vi "Routine.vi"(11 "TEMPLATE Queue in":refnum<class "TEMPLATE Queue.lvclass">) -> (3 "TEMPLATE Queue out":refnum<class "TEMPLATE Queue.lvclass">)   [LabVIEW 2021, in "_Template.lvlib" / "Templates.lvlib" / "TEMPLATE Queue.lvlib" / "TEMPLATE Queue.lvclass"]
uses:
  TEMPLATE Queue.lvclass
  TEMPLATE Queue.lvclass/TEMPLATE Queue.ctl
  <vilib>/Nathan Davis/jettl/jettl/Msg Strategy/Msg Strategy.lvclass
  <vilib>/Nathan Davis/jettl/jettl/Queue/Queue.lvclass
  C:/Program Files/National Instruments/LabVIEW 2021/vi.lib/Nathan Davis/jettl/jettl/jettl/jettl.lvclass
  C:/Program Files/National Instruments/LabVIEW 2021/vi.lib/Nathan Davis/jettl/Merge Error Msg Strategy/Merge Error/Merge Error.lvclass
  C:/Program Files/National Instruments/LabVIEW 2021/vi.lib/Nathan Davis/jettl/jettl/Queue/Queue.lvclass
  C:/Program Files/National Instruments/LabVIEW 2021/vi.lib/Nathan Davis/jettl/Create Event Msg Strategy/Create Event/Create Event.lvclass
  C:/Program Files/National Instruments/LabVIEW 2021/vi.lib/Nathan Davis/jettl/Create Queue Msg Strategy/Create Queue/Create Queue.lvclass
  C:/Program Files/National Instruments/LabVIEW 2021/vi.lib/Nathan Davis/jettl/jettl/Last Ack Created Event Msg Strategy/Last Ack Created Event/Last Ack Created Event.lvclass
  C:/Program Files/National Instruments/LabVIEW 2021/vi.lib/Nathan Davis/jettl/jettl/Last Ack Created Queue Msg Strategy/Last Ack Created Queue/Last Ack Created Queue.lvclass
  C:/Program Files/National Instruments/LabVIEW 2021/vi.lib/Nathan Davis/jettl/jettl/Last Ack Creator Queue Msg Strategy/Last Ack Creator Queue/Last Ack Creator Queue.lvclass
  C:/Program Files/National Instruments/LabVIEW 2021/vi.lib/Nathan Davis/jettl/Override Error Msg Strategy/Override Error/Override Error.lvclass
  C:/Program Files/National Instruments/LabVIEW 2021/vi.lib/Nathan Davis/jettl/Set Panel State Msg Strategy/Set Panel State/Set Panel State.lvclass
  C:/Program Files/National Instruments/LabVIEW 2021/vi.lib/Nathan Davis/jettl/Setup Msg Strategy/Setup/Setup.lvclass
  C:/Program Files/National Instruments/LabVIEW 2021/vi.lib/Nathan Davis/jettl/Teardown Msg Strategy/Teardown/Teardown.lvclass
  C:/git/jettl/jettl Tools/_Template/Templates/TEMPLATE Queue/TEMPLATE Queue/TEMPLATE Queue.lvclass
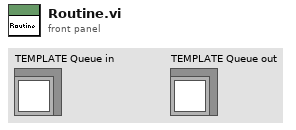
[diagram p1: front panel]
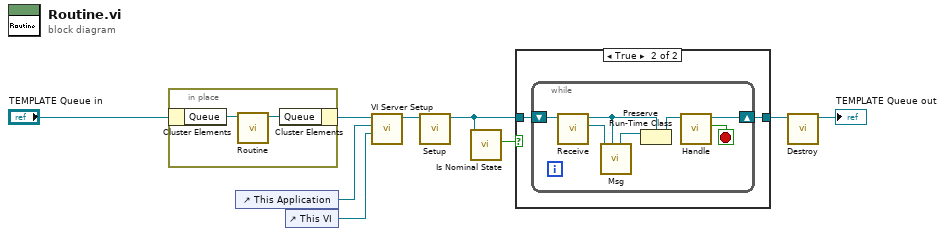
[diagram p0: block diagram]
diagram:
  n1 = in-place {
    n2 = in-place-cluster #1("TEMPLATE Queue in") -> ("Queue"=w11:refnum<class "Queue.lvclass">)
    n3 = call-dynamic "Routine.vi"("jettl in"=w11) -> ("jettl out"=w10:refnum<class "Queue.lvclass">)  [unwired: 10 in]
    n4 = in-place-cluster #1("Queue"=w10) -> (w4:refnum<class "TEMPLATE Queue.lvclass">)
  }
  n5 = control-ref of="This Application"() -> (w2:refnum<vi>)
  n6 = control-ref of="This VI"() -> (w1:refnum<vi>)
  n7 = call-dynamic "VI Server Setup.vi"("This VI"=w1, "This Application"=w2, "TEMPLATE Queue in"=w4) -> ("TEMPLATE Queue out"=w3:refnum<class "TEMPLATE Queue.lvclass">)  [unwired: 8 in]
  n8 = call-dynamic "Setup.vi"("TEMPLATE Queue in"=w3) -> ("TEMPLATE Queue out"=w6:refnum<class "TEMPLATE Queue.lvclass">)  [unwired: 10 in]
  n9 = call-dynamic "Is Nominal State.vi"("TEMPLATE Queue in"=w6) -> ("Is Nominal State?"=w5:bool)  [unwired: 10 in]
  n10 = case shown="True" w5 {
    tunnel: [w12 w14] -> w7
    tunnel: w6 -> [w12 w13]
    frame False {
    }
    frame True {
      n11 = while {
        shift-right: [w17] -> w14
        shift-left: w13 -> [w21]
        stop <- w16 stop-if-true
        n12 = call-dynamic "Receive.vi"("TEMPLATE Queue in"=w21) -> ("Msg Strategy"=w19:refnum<class "Msg Strategy.lvclass">, "TEMPLATE Queue out"=w18:refnum<class "TEMPLATE Queue.lvclass">)  [unwired: 9 in]
        n13 = call-dynamic "Msg.vi"("jettl in"=w18, "Msg Strategy in"=w19) -> ("jettl out"=w20:refnum<class "jettl.lvclass">)  [unwired: 9 in]
        n14 = Preserve Run-Time Class(object in=w20, 2:w18) -> (object out=w15:refnum<class "TEMPLATE Queue.lvclass">)  [unwired: 1 in, 1 out]
        n15 = call-dynamic "Handle.vi"("TEMPLATE Queue in"=w15) -> ("Destroy?"=w16:bool, "TEMPLATE Queue out"=w17:refnum<class "TEMPLATE Queue.lvclass">)  [unwired: 9 in]
      }
    }
  }
  n16 = call-dynamic "Destroy.vi"("TEMPLATE Queue in"=w7) -> ("TEMPLATE Queue out"=→"TEMPLATE Queue out":refnum<class "TEMPLATE Queue.lvclass">)  [unwired: 10 in]
